vi "Set Amplitude.vi"(8 "error in (no error)":errorcluster, 10 "Output amplitude":dbl=1.0 min=-1.0 max=1.0 format="%#_8pV", 11 "Red Pitaya Lock-in Driver in":refnum<class "Red Pitaya Lock-in Driver.lvclass">) -> (0 "error out":errorcluster, 3 "Red Pitaya Lock-in Driver out":refnum<class "Red Pitaya Lock-in Driver.lvclass">)   [LabVIEW 2021, in "Red Pitaya Lock-in Driver.lvclass"]
uses:
  Red Pitaya Lock-in Driver.lvclass
  Red Pitaya Lock-in Driver.lvclass/Red Pitaya Lock-in Driver.ctl
  RP Instrument/RP Instrument.lvclass
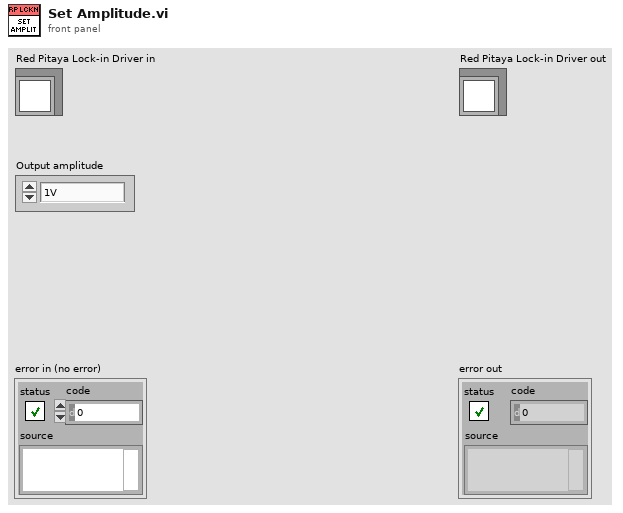
[diagram p1: front panel]
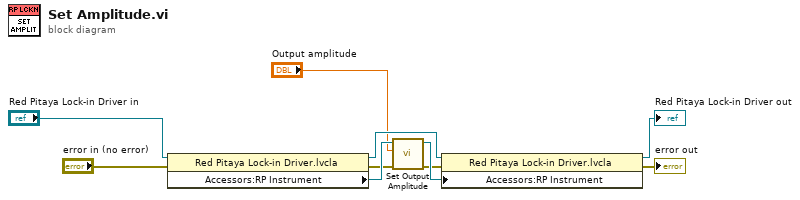
[diagram p0: block diagram]
diagram:
  n1 = property class="Red Pitaya Lock-in Driver.lvcla"(reference="Red Pitaya Lock-in Driver in", error in="error in (no error)") -> (reference out=w10:refnum<class "Red Pitaya Lock-in Driver.lvclass">, error out=w3:errorcluster, "Accessors:RP Instrument"=w9:refnum<class "RP Instrument.lvclass">)
  n2 = call-dynamic "Set Output Amplitude.vi"("error in (no error)"=w3, "Output amplitude"="Output amplitude", "RP Instrument in"=w9) -> ("error out"=w4:errorcluster, "RP Instrument out"=w8:refnum<class "RP Instrument.lvclass">)  [unwired: 7 in]
  n3 = property class="Red Pitaya Lock-in Driver.lvcla"(reference=w10, error in=w4, "Accessors:RP Instrument"=w8) -> (reference out=→"Red Pitaya Lock-in Driver out":refnum<class "Red Pitaya Lock-in Driver.lvclass">, error out=→"error out":errorcluster)
